vi "AutoFeed_Back.vi"(1 "Code 4":string, 2 "Error_4_En":bool, 4 "Code 3":string, 5 "Code 2":string, 6 "Error_3_En":bool, 7 "Error_2_En":bool, 8 "Code 1":string, 9 "Error_1_En":bool, 10 "Time (ms)":i32, 11 "State":dbl) -> (3 "Feedback_State":cluster{"Time_Met":bool, "error ":errorcluster})   [LabVIEW 2015]
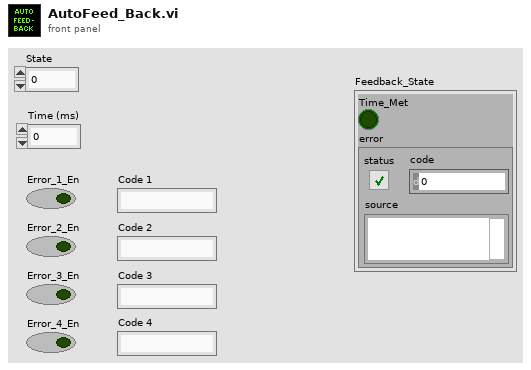
[diagram p1: front panel]
types:
  T1 = enum16{"Standard", "Momentary Falling", "Momentary Rising", "Momentary Falling and Rising"}
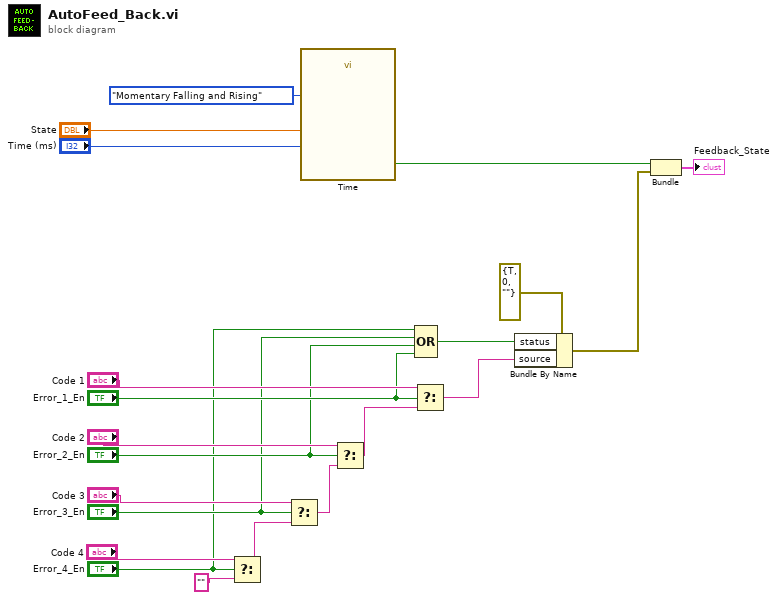
[diagram p0: block diagram]
diagram:
  n1 = Select(t="Code 4", s="Error_4_En", f="" ("source")) -> (s? t:f=w17:string)
  n2 = Select(t="Code 3", s="Error_3_En", f=w17) -> (s? t:f=w16:string)
  n3 = call "Time.vi"("Reset_Int"="State", "Configuration"=T1."Momentary Falling and Rising", "Time_Limit  (ms)"="Time (ms)") -> ("Time_Met"=w21:bool)  [unwired: 8 in]
  n4 = Select(t="Code 2", s="Error_2_En", f=w16) -> (s? t:f=w15:string)
  n5 = Compound Arithmetic op=OR("Error_4_En", "Error_3_En", "Error_2_En", "Error_1_En") -> (w4:bool)
  n6 = Select(t="Code 1", s="Error_1_En", f=w15) -> (s? t:f=w3:string)
  n7 = Bundle By Name(cluster=errorcluster {"status"=TRUE, "code"=0, "source"=""} ("error"), "status"=w4, "source"=w3) -> (w2:errorcluster)
  n8 = Bundle("Time_Met"=w21, "error"=w2) -> (→"Feedback_State":cluster{"Time_Met":bool, "error ":errorcluster})  [unwired: 1 in]
